vi "Do.vi"(8 "error in (no error)":cluster{"状态":bool, "代码":i32, "源":string} caption="错误输入（无错误）", 10 "操作者输入":refnum<class "Actor.lvclass">, 11 "冷却器更新水位消息":refnum<class "Cooler Update Water Level Msg.lvclass">) -> (0 "error out":cluster{"状态":bool, "代码":i32, "源":string} caption="错误输出", 2 "操作者输出":refnum<class "Actor.lvclass">)   [LabVIEW 2013, in "Evaporative Cooler.lvlib" / "Cooler Update Water Level Msg.lvclass"]
uses:
  Cooler Update Water Level Msg.lvclass
  <vilib>/ActorFramework/Actor/Actor.lvclass
  Evaporative Cooler/Evaporative Cooler.lvclass
  Water Level/Update Water Level Msg/Update Water Level Msg.lvclass/Update Water Level Msg.ctl
  Water Level/Update Water Level Msg/Update Water Level Msg.lvclass
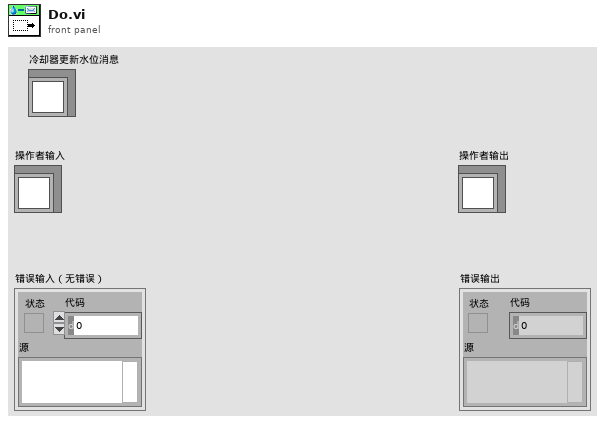
[diagram p1: front panel]
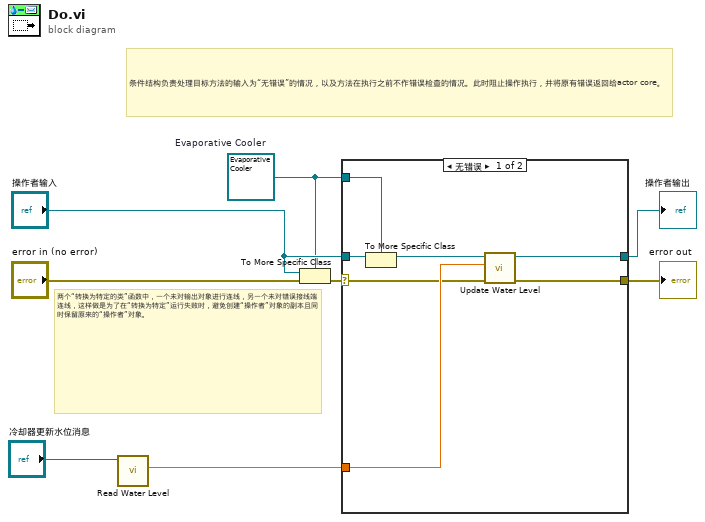
[diagram p0: block diagram]
diagram:
  w1 = refnum<class "Evaporative Cooler.lvclass"> refnum  # Evaporative Cooler
  # "两个“转换为特定的类”函数中，一个未对输出对象进行连线，另一个未对错误接线端连线，这样做是为了在“转换为特定”运行失败时，避免创建“操作者”对象的副本且同时保留原来的“操作者”对象。"
  # "条件结构负责处理目标方法的输入为“无错误”的情况，以及方法在执行之前不作错误检查的情况。此时阻止操作执行，并将原有错误返回给actor core。"
  n1 = call "Read Water Level.vi"("更新水位消息输入"="冷却器更新水位消息") -> ("水位"=w2:dbl)  [unwired: 9 in, 1 out]
  n2 = To More Specific Class(target class=w1, reference="操作者输入", error in="error in (no error)") -> (error out=w7:errorcluster)  [unwired: 1 out]
  n3 = case shown="无错误" w7 {
    selector: w7 -> [w9 w17]
    tunnel: [w11 w17] -> w6
    tunnel: [w12 w16] -> w5
    tunnel: "操作者输入" -> [w15 w16]
    tunnel: w1 -> [w14 _]
    tunnel: w2 -> [w10 _]
    frame No Error {
      n4 = To More Specific Class(target class=w14, reference=w15) -> (specific class reference=w13:refnum<class "Evaporative Cooler.lvclass">)  [unwired: 1 in, 1 out]
      n5 = call "Update Water Level.vi"("error in (no error)"=w9, "水位"=w10, "蒸发冷却器"=w13) -> ("error out"=w11:cluster{"状态":bool, "代码":i32, "源":string}, "蒸发冷却器"=w12:refnum<class "Evaporative Cooler.lvclass">)  [unwired: 7 in]
    }
    frame Error {
      # "如类型检查失败，则再次将原对象传出。"
    }
  }
  "error out" <- w6
  "操作者输出" <- w5
